vi "Find_Tote_Number_from_Pot.vi"(10 "On Bert?":bool=TRUE, 11 "Stack Clamp Angle":dbl format="%#_13g") -> (3 "Number of Totes":i8)   [LabVIEW 2014]
panel:
  in  "Ernie Range Number Cals":T1={"2 Tote"=153.0, "3 Tote"=172.0, "4 Tote"=192.0, "5 Tote "=211.0, "6 Tote "=220.0} {"6 Tote" format="%#_13g"; "5 Tote" format="%#_13g"; "4 Tote" format="%#_13g"; "3 Tote" format="%#_13g"; "2 Tote" format="%#_13g"}
  in  "Bert Range Number Cals":T1={"2 Tote"=141.0, "3 Tote"=162.0, "4 Tote"=180.0, "5 Tote "=200.0, "6 Tote "=215.0} {"6 Tote" format="%#_13g"; "5 Tote" format="%#_13g"; "4 Tote" format="%#_13g"; "3 Tote" format="%#_13g"; "2 Tote" format="%#_13g"}
  # "this is 5 totes"
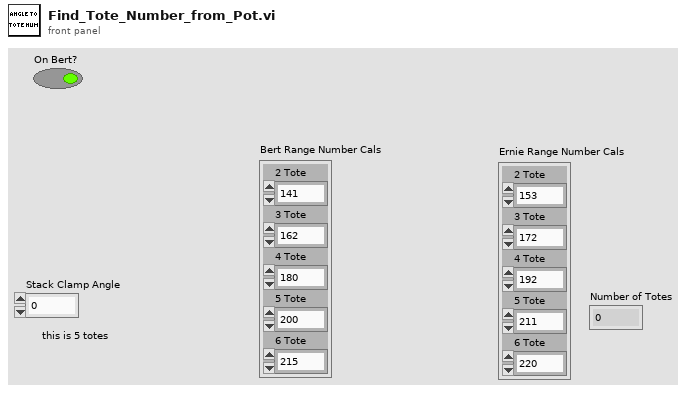
[diagram p1: front panel]
types:
  T1 = cluster{"2 Tote":dbl, "3 Tote":dbl, "4 Tote":dbl, "5 Tote ":dbl, "6 Tote ":dbl}
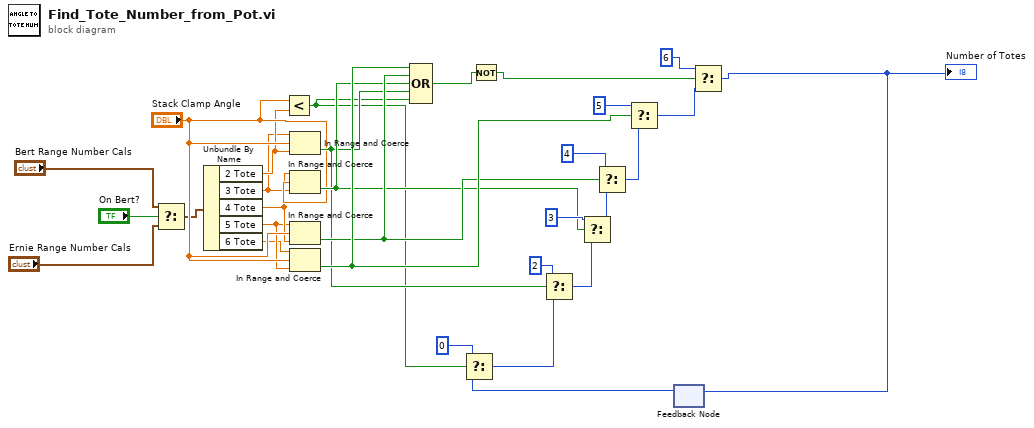
[diagram p0: block diagram]
diagram:
  n1 = Select(t="Bert Range Number Cals", s="On Bert?", f="Ernie Range Number Cals") -> (s? t:f=w1:T1)
  n2 = Unbundle By Name(w1) -> ("2 Tote"=w7:dbl, "3 Tote"=w6:dbl, "4 Tote"=w5:dbl, "5 Tote"=w4:dbl, "6 Tote"=w3:dbl)
  n3 = Less?(x="Stack Clamp Angle", y=w7) -> (x < y?=w13:bool)
  n4 = In Range and Coerce(upper limit=w6, x="Stack Clamp Angle", lower limit=w7) -> (In Range?=w14:bool)  [unwired: 1 out]
  n5 = In Range and Coerce(upper limit=w5, x="Stack Clamp Angle", lower limit=w6) -> (In Range?=w15:bool)  [unwired: 1 out]
  n6 = In Range and Coerce(upper limit=w4, x="Stack Clamp Angle", lower limit=w5) -> (In Range?=w16:bool)  [unwired: 1 out]
  n7 = In Range and Coerce(upper limit=w3, x="Stack Clamp Angle", lower limit=w4) -> (In Range?=w17:bool)  [unwired: 1 out]
  n8 = Compound Arithmetic op=OR(w17, w16, w15, w14, w13) -> (w12:bool)
  n9 = Not(x=w12) -> (.not. x?=w11:bool)
  n10 = feedback #1() -> (w23:i8)  [unwired: 1 in]
  n11 = Select(t=i8 0 ("Number of Totes 2"), s=w13, f=w23) -> (s? t:f=w18:i8)
  n12 = Select(t=i8 2 ("Number of Totes 2"), s=w14, f=w18) -> (s? t:f=w22:i8)
  n13 = Select(t=i8 3 ("Number of Totes 2"), s=w15, f=w22) -> (s? t:f=w21:i8)
  n14 = Select(t=i8 4 ("Number of Totes 2"), s=w16, f=w21) -> (s? t:f=w20:i8)
  n15 = Select(t=i8 5 ("Number of Totes 2"), s=w17, f=w20) -> (s? t:f=w19:i8)
  n16 = Select(t=i8 6 ("Number of Totes 2"), s=w11, f=w19) -> (s? t:f=w24:i8)
  "Number of Totes" <- w24
  n17 = feedback-in #1(w24) -> ()
